vi "Read Attributes.vi"(11 "Set DER SetPointQ Msg":refnum<class "Set DER SetPointQ Msg.lvclass">) -> (2 "Payload":cluster{"DER_SetPointQ":T1})   [LabVIEW 2018, in "Device Communication and Control Abstract Actor.lvlib" / "Set DER SetPointQ Msg.lvclass"]
uses:
  Set DER SetPointQ Msg.lvclass
  <vilib>/ORNL/CSEISMIC DDS/CSEISMIC DDS Base/Data Types/DER_SetPointQ.ctl
  <vilib>/ORNL/CSEISMIC DDS/CSEISMIC DDS Base/Data Types/Controls/DeviceID.ctl
  Set DER SetPointQ Msg.lvclass/Set DER SetPointQ Msg.ctl
  <vilib>/ORNL/CSEISMIC DDS/CSEISMIC DDS Base/CSEISMIC DDS.lvclass
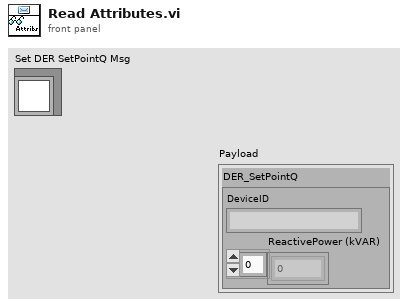
[diagram p1: front panel]
types:
  T1 = typedef "CSEISMIC DDS.lvlib/CSEISMIC DDS.lvclass/DER_SetPointQ.ctl" = cluster{"DeviceID":T2, "ReactivePower (kVAR)":dbl[]}
  T2 = typedef "CSEISMIC DDS.lvlib/CSEISMIC DDS.lvclass/DeviceID.ctl" = string
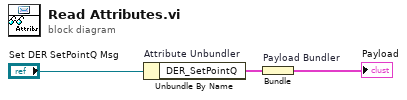
[diagram p0: block diagram]
diagram:
  n1 = Unbundle By Name "Attribute Unbundler"("Set DER SetPointQ Msg") -> ("DER_SetPointQ"=w1:T1)
  n2 = Bundle "Payload Bundler"("DER_SetPointQ"=w1) -> (→"Payload":cluster{"DER_SetPointQ":T1})  [unwired: 1 in]
